vi "16BitDisplayMapping2.vi"(3 "Image":T2, 4 "BitDepth":u32, 5 "ImageType":T1 items=["Grayscale (U8)", "Grayscale (I16)", "Grayscale (SGL)", "Complex (CSG)", "RGB (U32)", "HSL (U32)", "RGB (U64)", "Grayscale (U16)"], 6 "DisplayMappingInput":T3) -> (1 "OK":bool, 2 "DisplayMappingOutput":T3)   [LabVIEW 2009]
uses:
  <vilib>/vision/Image Controls.llb/IMAQ Image.ctl
panel:
  out "Not 16-bit String":string="16-Bit Image Not Available"
  in  "OldValue":bool caption="Apply mapping only when Configured Bit Depth is 0"
  out "FullDynamic":string="Using the full dynamic range"
  out "MSB":u32 caption="MSB:"
  out "LSB":u32 caption="LSB:"
  out "Configured Bit Depth":u32 caption="Configured Bit Depth:"
  in  "Percentage Range":cluster{"Min":i32, "Min":i32}(slide)={"Min"=0, "Min"=128} scale=0.0..100.0
  in  "Shift Value":i32(slide)=8 caption="# Shifts:" scale=8.0..0.0
  in  "Range":cluster{"Min":i32, "Min":i32}(slide)={"Min"=0, "Min"=128} scale=-32768.0..32767.0
  in  "Conversion Method":u32(ring) items=["Default"=10, "Most Significant Bits"=11, "Full Dynamic"=12, "Downshift"=13, "Given Range"=14, "90% Dynamic"=15, "Given Percent Range"=16]
  in  "Cancel":bool
  in  "OK":bool
  out "Preview":T2(plugin-control)
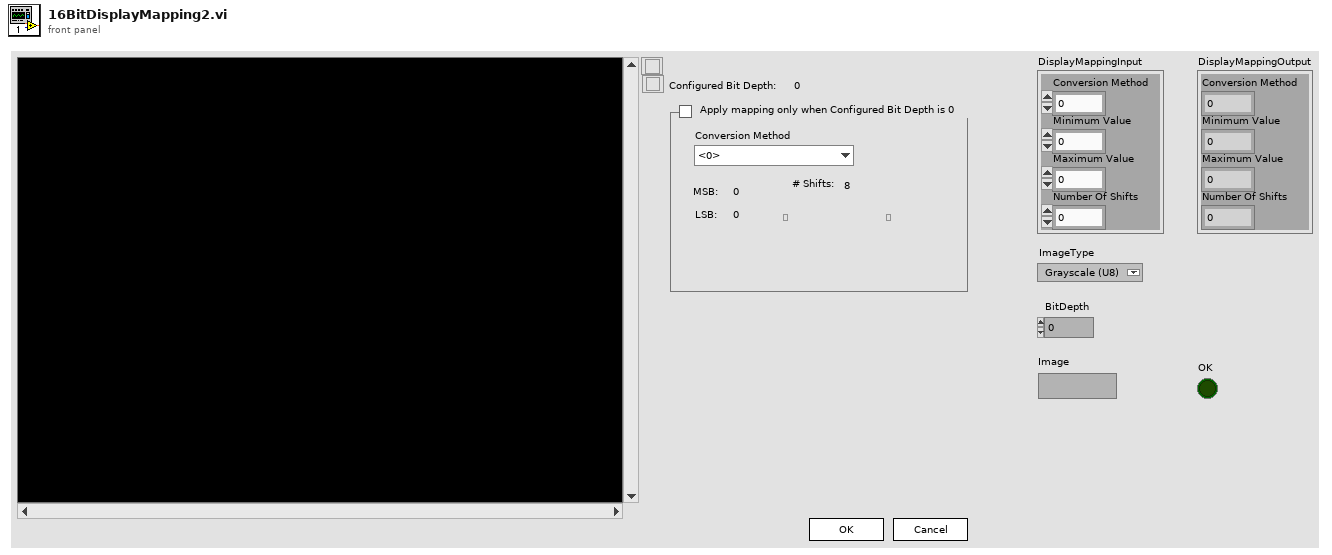
[diagram p1: front panel]
types:
  T1 = typedef "Image Type" = u32
  T2 = typedef "IMAQ Image.ctl" = refnum<image>
  T3 = cluster{"Conversion Method":u32, "Minimum Value":i32, "Maximum Value":i32, "Number Of Shifts":i32}
  T4 = cluster{"Minimum Value":i32, "Maximum Value":i32}
  T5 = enum32{"Invalid", "Standard", "Closed", "Hidden", "Minimized", "Maximized"}
  T6 = cluster{"Conversion Method":u32, "Min":i32, "Min":i32, "Number Of Shifts":i32}
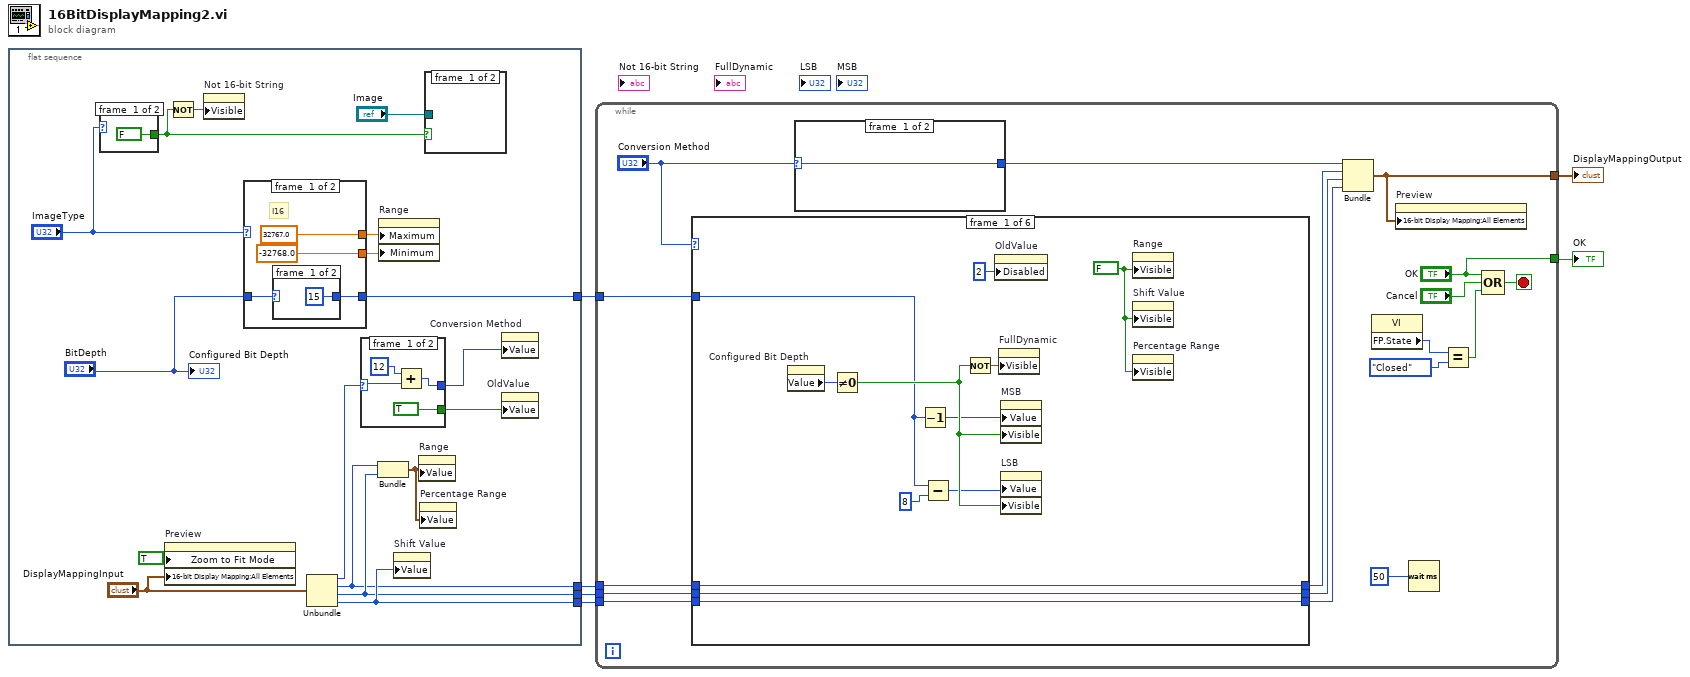
[diagram p0: block diagram]
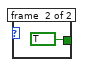
[diagram p2: hidden frame]
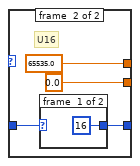
[diagram p4: hidden frame]
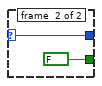
[diagram p6: hidden frame]
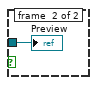
[diagram p7: hidden frame]
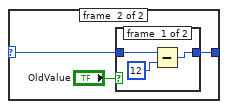
[diagram p8: hidden frame]
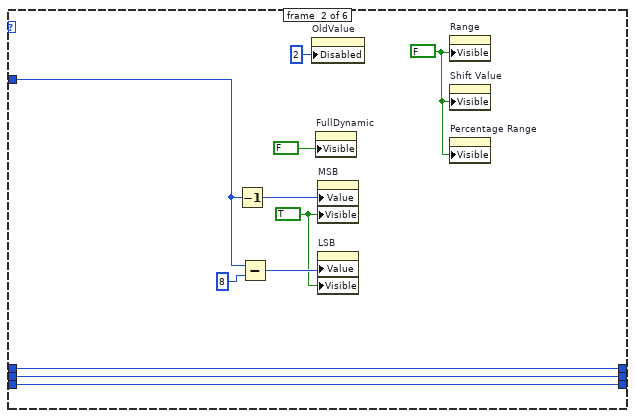
[diagram p10: hidden frame]
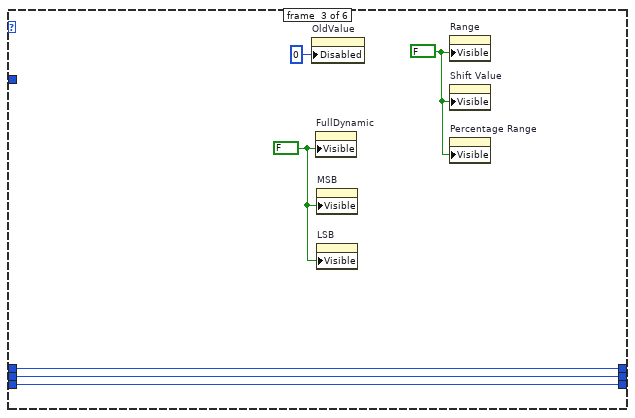
[diagram p11: hidden frame]
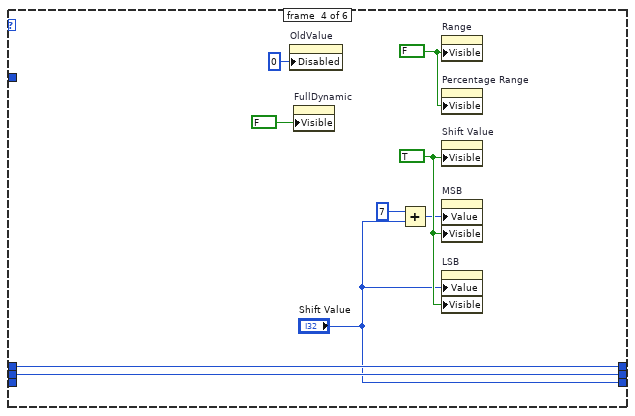
[diagram p12: hidden frame]
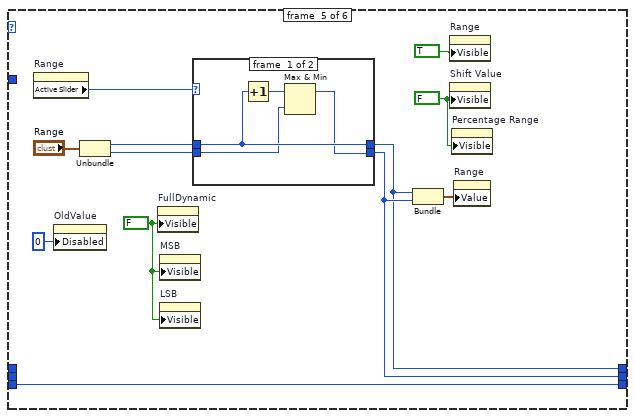
[diagram p13: hidden frame]
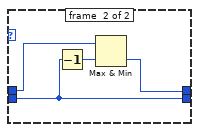
[diagram p14: hidden frame]
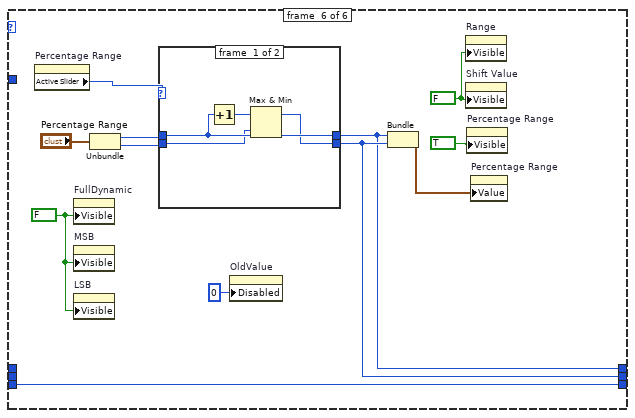
[diagram p15: hidden frame]
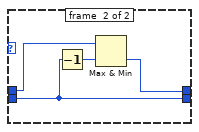
[diagram p16: hidden frame]
diagram:
  n1 = flat-sequence {
    tunnel: [w21] -> w4
    tunnel: [w20] -> w3
    tunnel: [w18] -> w2
    tunnel: [w12] -> w1
    frame #0 {
      n2 = case shown="1, 7" "ImageType" {
        tunnel: [FALSE ("x") TRUE ("x")] -> w9
        frame #0 {
        }
        frame #1 {
        }
      }
      n3 = property on="Preview" class="ImageControl"("Zoom to Fit Mode"=TRUE, "16-bit Display Mapping:All Elements"="DisplayMappingInput") -> ()  [unwired: 2 in, 2 out]
      n4 = Not(x=w9) -> (.not. x?=w23:bool)
      n5 = property on="Not 16-bit String" class="String"("Visible"=w23) -> ()  [unwired: 2 in, 2 out]
      n6 = case shown="7" "ImageType" {
        tunnel: [32767.0 ("Data Range:Maximum") 65535.0 ("Data Range:Maximum")] -> w14
        tunnel: [-32768.0 ("Data Range:Minimum") 0.0 ("Data Range:Minimum")] -> w13
        tunnel: "BitDepth" -> [w26 w33]
        tunnel: [w27 w32] -> w12
        frame #0 {
          # "I16"
          n7 = case shown="1, Default" w26 {
            selector: w26 -> [_ w31]
            tunnel: [u32 15 ("Bit Depth") w31] -> w27
            frame #0 {
            }
            frame #1 {
            }
          }
        }
        frame #1 {
          # "U16"
          n8 = case shown="0" w33 {
            selector: w33 -> [_ w37]
            tunnel: [u32 16 ("Bit Depth") w37] -> w32
            frame #0 {
            }
            frame #1 {
            }
          }
        }
      }
      n9 = Unbundle("DisplayMappingInput") -> ("Conversion Method"=w8:u32, "Minimum Value"=w18:i32, "Maximum Value"=w20:i32, "Number Of Shifts"=w21:i32)
      n10 = case shown="10..16, Default" w8 {
        selector: w8 -> [w40 w43]
        tunnel: [w41 w43] -> w16
        tunnel: [TRUE ("OldValue") FALSE ("OldValue")] -> w17
        frame #0 {
          n11 = Add(x=12, y=w40) -> (x+y=w41:u32)
        }
        frame #1 {
        }
      }
      n12 = Bundle("Minimum Value"=w18, "Maximum Value"=w20) -> (w19:T4)  [unwired: 1 in]
      n13 = property on="Range" class="Slide (strict)"("Maximum"=w14, "Minimum"=w13) -> ()  [unwired: 2 in, 2 out]
      n14 = property on="Shift Value" class="Slide (strict)"("Value"=w21) -> ()  [unwired: 2 in, 2 out]
      n15 = property on="Range" class="Slide (strict)"("Value"=w19) -> ()  [unwired: 2 in, 2 out]
      n16 = property on="Percentage Range" class="Slide (strict)"("Value"=w19) -> ()  [unwired: 2 in, 2 out]
      n17 = case shown="True" w9 {
        tunnel: "Image" -> [_ w44]
        frame #0 {
        }
        frame #1 {
          "Preview" <- w44
        }
      }
      n18 = property on="Conversion Method" class="Ring (strict)"("Value"=w16) -> ()  [unwired: 2 in, 2 out]
      n19 = property on="OldValue" class="Bool (strict)"("Value"=w17) -> ()  [unwired: 2 in, 2 out]
      "Configured Bit Depth" <- "BitDepth"
    }
  }
  n20 = while {
    tunnel: ["OK"] -> w5
    tunnel: [w57] -> w6
    tunnel: w2 -> [w56]
    tunnel: w3 -> [w55]
    tunnel: w4 -> [w54]
    tunnel: w1 -> [w47]
    stop <- w60 stop-if-true
    n21 = case shown="10, Default" "Conversion Method" {
      tunnel: [w81 w92 w98 w106 w110 w130] -> w52
      tunnel: w56 -> [w81 w92 w98 w106 _ _]
      tunnel: [w80 w91 w97 w107 w111 w131] -> w51
      tunnel: w55 -> [w80 w91 w97 w107 _ _]
      tunnel: [w79 w90 w96 "Shift Value" w119 w139] -> w53
      tunnel: w54 -> [w79 w90 w96 _ w119 w139]
      tunnel: w47 -> [w71 w85 _ _ _ _]
      frame #0 {
        w78 = FALSE ("Visible")
        n22 = property on="Configured Bit Depth" class="DigNum (strict)"() -> ("Value"=w76:u32)  [unwired: 2 in, 2 out]
        n23 = Not Equal To 0?(x=w76) -> (x != 0?=w74:bool)
        n24 = Decrement(x=w71) -> (x-1=w73:u32)
        n25 = Subtract(x=w71, y=u32 8) -> (x-y=w72:u32)
        n26 = Not(x=w74) -> (.not. x?=w75:bool)
        n27 = property on="OldValue" class="Bool (strict)"("Disabled"=u8 2) -> ()  [unwired: 2 in, 2 out]
        n28 = property on="FullDynamic" class="Str"("Visible"=w75) -> ()  [unwired: 2 in, 2 out]
        n29 = property on="MSB" class="DigNum (strict)"("Value"=w73, "Visible"=w74) -> ()  [unwired: 2 in, 2 out]
        n30 = property on="LSB" class="DigNum (strict)"("Value"=w72, "Visible"=w74) -> ()  [unwired: 2 in, 2 out]
        n31 = property on="Range" class="Slide (strict)"("Visible"=w78) -> ()  [unwired: 2 in, 2 out]
        n32 = property on="Shift Value" class="Slide (strict)"("Visible"=w78) -> ()  [unwired: 2 in, 2 out]
        n33 = property on="Percentage Range" class="Slide (strict)"("Visible"=w78) -> ()  [unwired: 2 in, 2 out]
      }
      frame #1 {
        w82 = TRUE ("Visible")
        w89 = FALSE ("Visible")
        n34 = Decrement(x=w85) -> (x-1=w87:u32)
        n35 = Subtract(x=w85, y=u32 8) -> (x-y=w86:u32)
        n36 = property on="OldValue" class="Bool (strict)"("Disabled"=u8 2) -> ()  [unwired: 2 in, 2 out]
        n37 = property on="FullDynamic" class="Str"("Visible"=FALSE) -> ()  [unwired: 2 in, 2 out]
        n38 = property on="MSB" class="DigNum (strict)"("Value"=w87, "Visible"=w82) -> ()  [unwired: 2 in, 2 out]
        n39 = property on="LSB" class="DigNum (strict)"("Value"=w86, "Visible"=w82) -> ()  [unwired: 2 in, 2 out]
        n40 = property on="Range" class="Slide (strict)"("Visible"=w89) -> ()  [unwired: 2 in, 2 out]
        n41 = property on="Shift Value" class="Slide (strict)"("Visible"=w89) -> ()  [unwired: 2 in, 2 out]
        n42 = property on="Percentage Range" class="Slide (strict)"("Visible"=w89) -> ()  [unwired: 2 in, 2 out]
      }
      frame #2 {
        w93 = FALSE ("Visible")
        w95 = FALSE ("Visible")
        n43 = property on="OldValue" class="Bool (strict)"("Disabled"=u8 0) -> ()  [unwired: 2 in, 2 out]
        n44 = property on="FullDynamic" class="Str"("Visible"=w93) -> ()  [unwired: 2 in, 2 out]
        n45 = property on="MSB" class="DigNum (strict)"("Visible"=w93) -> ()  [unwired: 2 in, 2 out]
        n46 = property on="LSB" class="DigNum (strict)"("Visible"=w93) -> ()  [unwired: 2 in, 2 out]
        n47 = property on="Range" class="Slide (strict)"("Visible"=w95) -> ()  [unwired: 2 in, 2 out]
        n48 = property on="Shift Value" class="Slide (strict)"("Visible"=w95) -> ()  [unwired: 2 in, 2 out]
        n49 = property on="Percentage Range" class="Slide (strict)"("Visible"=w95) -> ()  [unwired: 2 in, 2 out]
      }
      frame #3 {
        w104 = TRUE ("Visible")
        w105 = FALSE ("Visible")
        n50 = property on="OldValue" class="Bool (strict)"("Disabled"=u8 0) -> ()  [unwired: 2 in, 2 out]
        n51 = property on="FullDynamic" class="Str"("Visible"=FALSE) -> ()  [unwired: 2 in, 2 out]
        n52 = Add(x=7, y="Shift Value") -> (x+y=w103:i32)
        n53 = property on="Range" class="Slide (strict)"("Visible"=w105) -> ()  [unwired: 2 in, 2 out]
        n54 = property on="Percentage Range" class="Slide (strict)"("Visible"=w105) -> ()  [unwired: 2 in, 2 out]
        n55 = property on="Shift Value" class="Slide (strict)"("Visible"=w104) -> ()  [unwired: 2 in, 2 out]
        n56 = property on="MSB" class="DigNum (strict)"("Value"=w103, "Visible"=w104) -> ()  [unwired: 2 in, 2 out]
        n57 = property on="LSB" class="DigNum (strict)"("Value"="Shift Value", "Visible"=w104) -> ()  [unwired: 2 in, 2 out]
      }
      frame #4 {
        w108 = FALSE ("Visible")
        w117 = FALSE ("Visible")
        n58 = property on="Range" class="Slide (strict)"() -> ("Active Slider"=w116:i32)  [unwired: 2 in, 2 out]
        n59 = property on="OldValue" class="Bool (strict)"("Disabled"=u8 0) -> ()  [unwired: 2 in, 2 out]
        n60 = Unbundle("Range") -> ("Min"=w114:i32, "Min"=w113:i32)
        n61 = property on="FullDynamic" class="Str"("Visible"=w108) -> ()  [unwired: 2 in, 2 out]
        n62 = property on="MSB" class="DigNum (strict)"("Visible"=w108) -> ()  [unwired: 2 in, 2 out]
        n63 = property on="LSB" class="DigNum (strict)"("Visible"=w108) -> ()  [unwired: 2 in, 2 out]
        n64 = case shown="1" w116 {
          tunnel: w114 -> [w123 w125]
          tunnel: w113 -> [w122 w127]
          tunnel: [w123 w126] -> w110
          tunnel: [w121 w127] -> w111
          frame #0 {
            n65 = Increment(x=w123) -> (x+1=w120:i32)
            n66 = Max & Min(x=w120, y=w122) -> (max(x,y)=w121:i32)  [unwired: 1 out]
          }
          frame #1 {
            n67 = Decrement(x=w127) -> (x-1=w124:i32)
            n68 = Max & Min(x=w125, y=w124) -> (min(x,y)=w126:i32)  [unwired: 1 out]
          }
        }
        n69 = Bundle("Min"=w110, "Min"=w111) -> (w112:cluster{"Min":i32, "Min":i32})  [unwired: 1 in]
        n70 = property on="Range" class="Slide (strict)"("Visible"=TRUE) -> ()  [unwired: 2 in, 2 out]
        n71 = property on="Shift Value" class="Slide (strict)"("Visible"=w117) -> ()  [unwired: 2 in, 2 out]
        n72 = property on="Percentage Range" class="Slide (strict)"("Visible"=w117) -> ()  [unwired: 2 in, 2 out]
        n73 = property on="Range" class="Slide (strict)"("Value"=w112) -> ()  [unwired: 2 in, 2 out]
      }
      frame #5 {
        w128 = FALSE ("Visible")
        w137 = FALSE ("Visible")
        n74 = property on="Percentage Range" class="Slide (strict)"() -> ("Active Slider"=w133:i32)  [unwired: 2 in, 2 out]
        n75 = property on="FullDynamic" class="Str"("Visible"=w128) -> ()  [unwired: 2 in, 2 out]
        n76 = property on="MSB" class="DigNum (strict)"("Visible"=w128) -> ()  [unwired: 2 in, 2 out]
        n77 = property on="LSB" class="DigNum (strict)"("Visible"=w128) -> ()  [unwired: 2 in, 2 out]
        n78 = Unbundle("Percentage Range") -> ("Min"=w135:i32, "Min"=w134:i32)
        n79 = case shown="0, Default" w133 {
          tunnel: w135 -> [w143 w145]
          tunnel: w134 -> [w142 w147]
          tunnel: [w143 w146] -> w130
          tunnel: [w141 w147] -> w131
          frame #0 {
            n80 = Increment(x=w143) -> (x+1=w140:i32)
            n81 = Max & Min(x=w140, y=w142) -> (max(x,y)=w141:i32)  [unwired: 1 out]
          }
          frame #1 {
            n82 = Decrement(x=w147) -> (x-1=w144:i32)
            n83 = Max & Min(x=w145, y=w144) -> (min(x,y)=w146:i32)  [unwired: 1 out]
          }
        }
        n84 = property on="OldValue" class="Bool (strict)"("Disabled"=u8 0) -> ()  [unwired: 2 in, 2 out]
        n85 = Bundle("Min"=w130, "Min"=w131) -> (w132:cluster{"Min":i32, "Min":i32})  [unwired: 1 in]
        n86 = property on="Range" class="Slide (strict)"("Visible"=w137) -> ()  [unwired: 2 in, 2 out]
        n87 = property on="Shift Value" class="Slide (strict)"("Visible"=w137) -> ()  [unwired: 2 in, 2 out]
        n88 = property on="Percentage Range" class="Slide (strict)"("Visible"=TRUE) -> ()  [unwired: 2 in, 2 out]
        n89 = property on="Percentage Range" class="Slide (strict)"("Value"=w132) -> ()  [unwired: 2 in, 2 out]
      }
    }
    n90 = case shown="12..16" "Conversion Method" {
      selector: "Conversion Method" -> [w62 w63]
      tunnel: [w62 w64] -> w46
      frame #0 {
      }
      frame #1 {
        n91 = case shown="True" "OldValue" {
          tunnel: [w67 w69] -> w64
          tunnel: w63 -> [w66 w69]
          frame #0 {
            n92 = Subtract(x=w66, y=12 ("x")) -> (x-y=w67:u32)
          }
          frame #1 {
          }
        }
      }
    }
    n93 = Bundle("Conversion Method"=w46, "Min"=w52, "Min"=w51, "Number Of Shifts"=w53) -> (w57:T6)  [unwired: 1 in]
    n94 = property class="VI"() -> ("FP.State"=w50:T5)  [unwired: 2 in, 2 out]
    n95 = property on="Preview" class="ImageControl"("16-bit Display Mapping:All Elements"=w57) -> ()  [unwired: 2 in, 2 out]
    n96 = Wait (ms)(milliseconds to wait=u32 50) -> ()  [unwired: 1 out]
    n97 = Equal?(x=w50, y=T5."Closed") -> (x = y?=w48:bool)
    n98 = Compound Arithmetic op=OR("OK", "Cancel", w48) -> (w60:bool)
  }
  "DisplayMappingOutput" <- w6
  "OK" <- w5
